vi "DAQmx - Read Accele Data_SubVIs-某型振动实验台测试系统.vi"(8 "Error In":errorcluster, 9 "Buffer":u16[](array[numeric]), 10 "pDMAStatus":i32[](array[numeric]), 11 "task in":T1={"Task Info"={"Accele Task"=[], "Simulate"=FALSE, "采样率"={"AISampleRate"=10123, "CouplingType"=10000, "Butter"=1000}, "Trig"={"PreTrigCNT"=0, "TriggerMode"=enum."中间触发", "TriggerSource"=enum."软件触发", "ATRTriggerChannel"=enum."通道0", "TriggerDir"=enum."下降沿触发", "TrigLevelVolt"=0.0, "bAvailableTrig"=FALSE}, "clock"={"EN"=FALSE, "clocksource"=enum."内部时钟", "outclocksource"=enum."Trig0"}, "delay(S)"=0.0}, "datain"={"nSegmentCount"=0, "chaneldataSize"=8192, "t0 in"=timestamp(0 s since 1904-01-01), "nsegmentsize"=0, "chanelcouter"=0}, "times"=0.0, "timer"=[], "\nen"=FALSE} {"Task Info"."采样率"."CouplingType" items=["直流耦合", "交流耦合"]}) -> (0 "Error Out":errorcluster, 1 "Data":waveform(dbl)[](array[waveform]), 2 "pDMAStatus out":i32[](array[numeric]), 3 "task out":T1={"Task Info"={"Accele Task"=[], "Simulate"=FALSE, "采样率"={"AISampleRate"=10123, "CouplingType"=10000, "Butter"=1000}, "Trig"={"PreTrigCNT"=0, "TriggerMode"=enum."中间触发", "TriggerSource"=enum."软件触发", "ATRTriggerChannel"=enum."通道0", "TriggerDir"=enum."下降沿触发", "TrigLevelVolt"=0.0, "bAvailableTrig"=FALSE}, "clock"={"EN"=FALSE, "clocksource"=enum."内部时钟", "outclocksource"=enum."Trig0"}, "delay(S)"=0.0}, "datain"={"nSegmentCount"=0, "chaneldataSize"=8192, "t0 in"=timestamp(0 s since 1904-01-01), "nsegmentsize"=0, "chanelcouter"=0}, "times"=0.0, "timer"=[], "\nen"=FALSE} {"Task Info"."采样率"."CouplingType" items=["直流耦合", "交流耦合"]})   [LabVIEW 2009]
doc: "读取振动数据"
uses:
  Ctrls/Acceleration Channel Config_Ctrls-某型振动实验台测试系统.ctl
  Ctrls/Sample Information.ctl
  Ctrls/Task Info.ctl
  Ctrls/Trig.ctl
  Ctrls/clock.ctl
  Ctrls/DATA info.ctl
  Ctrls/task.ctl
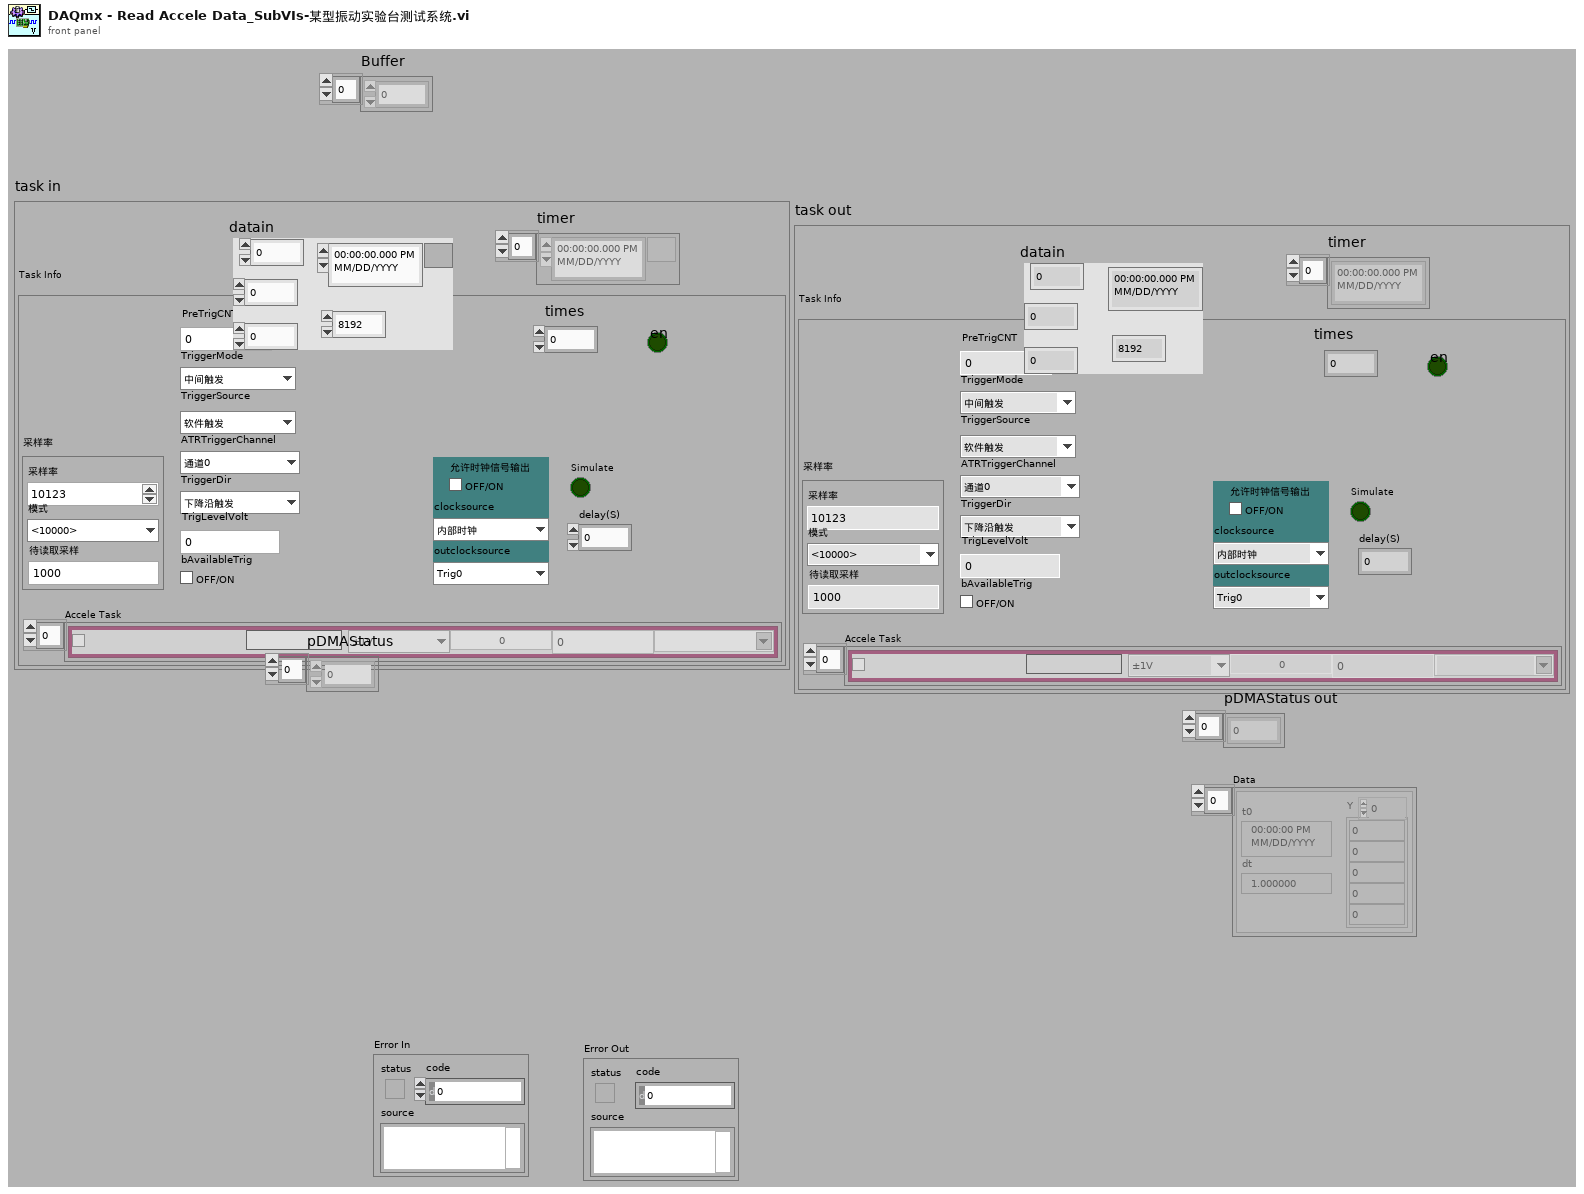
[diagram p1: front panel]
types:
  T1 = typedef "task.ctl" = cluster{"Task Info":T2, "datain":T7, "times":dbl, "timer":timestamp[], "\nen":bool}
  T2 = typedef "Task Info.ctl" = cluster{"Accele Task":T3[], "Simulate":bool, "采样率":T4, "Trig":T5, "clock":T6, "delay(S)":dbl}
  T3 = typedef "Acceleration Channel Config_Ctrls-某型振动实验台测试系统.ctl" = cluster{"Enable":bool, "Name":string, "range":enum16{"±1V", "±5V"}, "SensValue":dbl, "PhysicalName":string, "off":dbl, "Sensunits":string}
  T4 = typedef "Sample Information.ctl" = cluster{"AISampleRate":i32, "CouplingType":i32, "Butter":i32}
  T5 = typedef "Trig.ctl" = cluster{"PreTrigCNT":i32, "TriggerMode":enum16{"中间触发", "后触发", "预触发", "硬件延时触发"}, "TriggerSource":enum16{"软件触发", "DTR信号源", "ATR信号源", "Triger信号触发"}, "ATRTriggerChannel":enum16{"通道0", "通道1", "通道2", "通道3"}, "TriggerDir":enum16{"下降沿触发", "上升沿触发", "上下边没均触发"}, "TrigLevelVolt":sgl, "bAvailableTrig":bool}
  T6 = typedef "clock.ctl" = cluster{"EN":bool, "clocksource":enum16{"内部时钟", "外部时钟"}, "outclocksource":enum16{"Trig0", "Trig1", "Trig2", "Trig3", "Trig4", "Trig5", "Trig6", "Trig7", "PXI_STAR"}}
  T7 = typedef "DATA info.ctl" = cluster{"nSegmentCount":i32, "chaneldataSize":i32, "t0 in":timestamp, "nsegmentsize":i32, "chanelcouter":i32}
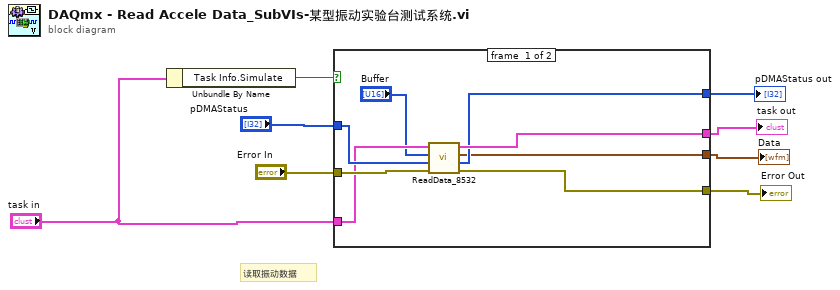
[diagram p0: block diagram]
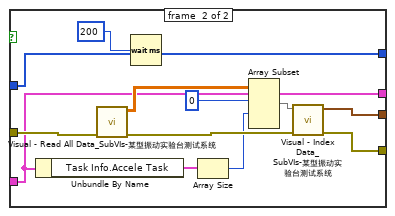
[diagram p2: hidden frame]
diagram:
  # "读取振动数据"
  n1 = Unbundle By Name("task in") -> ("Task Info.Simulate"=w1:bool)
  n2 = case shown="假" w1 {
    tunnel: "Error In" -> [w16 w28]
    tunnel: [w15 w26] -> w7
    tunnel: [w12 w25] -> w8
    tunnel: "task in" -> [w10 w17]
    tunnel: [w14 w17] -> w5
    tunnel: [w13 w18] -> w4
    tunnel: "pDMAStatus" -> [w11 w18]
    frame #0 {
      n3 = call "ReadData_8532.vi"("error in (no error)"=w16, "pDMAStatus"=w11, "Buffer"="Buffer", "task"=w10) -> ("error out"=w15:errorcluster, "pDMAStatus out"=w13:i32[], "Data"=w12:waveform(dbl)[], "task out"=w14:T1)  [unwired: 4 out]
    }
    frame #1 {
      n4 = Unbundle By Name(w17) -> ("Task Info.Accele Task"=w20:T3[])
      n5 = call "Visual - Read All Data_SubVIs-某型振动实验台测试系统.vi"("error in"=w28) -> ("error out"=w27:errorcluster, "Data"=w22:dbl[][])  [unwired: 1 in, 8 out]
      n6 = Wait (ms)(milliseconds to wait=u32 200) -> ()  [unwired: 1 out]
      n7 = Array Size(array=w20) -> (size(s)=w19:i32)
      n8 = Array Subset(array=w22, index (row)=0 ("index"), length (row)=w19) -> (w21:dbl[][])  [unwired: 2 in]
      n9 = call "Visual - Index Data_SubVIs-某型振动实验台测试系统.vi"("Error In"=w27, "Data"=w21) -> ("Error Out"=w26:errorcluster, "Data"=w25:waveform(dbl)[])  [unwired: 1 in, 7 out]
    }
  }
  "Data" <- w8
  "Error Out" <- w7
  "task out" <- w5
  "pDMAStatus out" <- w4
